vi "Insert an Empty Slot.vi"   [LabVIEW 2019]
doc: "Inserts an empty slot into an existing palette."
uses:
  <vilib>/Palette API/Palette Menu/Public Type Define/Palette type.ctl
  <vilib>/Palette API/Palette Menu/Public Type Define/Item.ctl
  <vilib>/Palette API/Palette Menu/Palette Menu.lvlib
panel:
  # "Overview: Demonstrates the use of the Palette Editing VIs to add an empty slot to an existing palette.\nInstructions:\n1. Make sure you have already run the Create New Palette.vi example.\n2. Run this VI. It will add an empty slot in the second position of the Functions > User Libraries > Palette API. See the block diagram for more information."
types:
  T1 = typedef "Palette Menu.lvlib/Palette type.ctl" = i32
  T2 = typedef "Palette Menu.lvlib/Palette Data.ctl" = cluster{"display name":string, "view format":T3, "palette width":i16, "items":T4, "256 color icon":picture, "B&W color icon":picture, "help information":T6, "palette description":string, "synchronize information":T7}
  T3 = typedef "Palette Menu.lvlib/View Format.ctl" = u16
  T4 = typedef "Palette Menu.lvlib/Items.ctl" = T5[]
  T5 = typedef "Palette Menu.lvlib/Item.ctl" = cluster{"item path":path, "library path":path, "use default lvlib palette":bool, "short name":string, "place VI contents":bool, "hide synchronized item":bool, "reserve spot for synch item":bool, "configure when placing VI contents":bool}
  T6 = typedef "Palette Menu.lvlib/Help Info.ctl" = cluster{"help tag":string, "help file path ":path}
  T7 = typedef "Palette Menu.lvlib/Synchronize Info.ctl" = cluster{"synchronize with directory":bool, "synchronize directory path":path}
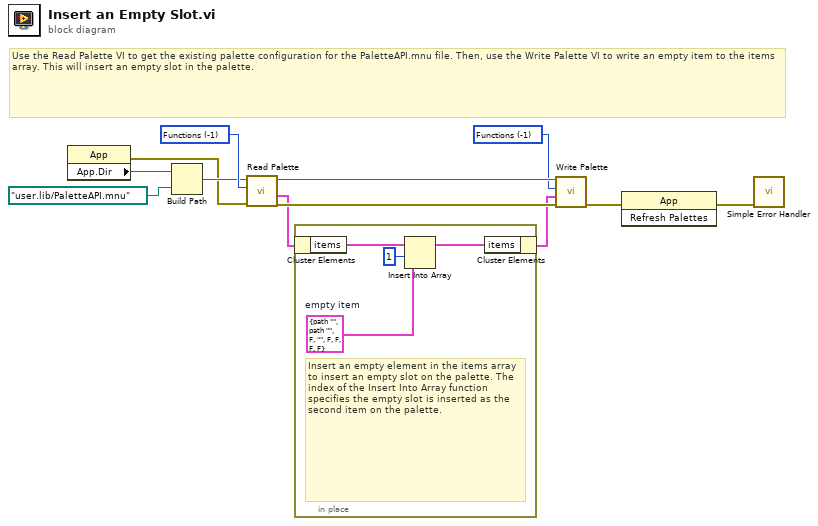
[diagram p0: block diagram]
diagram:
  w2 = T1 -1 items=["Functions"=-1, "Controls"=-2] ("palette type")
  w11 = T1 -1 items=["Functions"=-1, "Controls"=-2] ("palette type")
  # "Use the Read Palette VI to get the existing palette configuration for the PaletteAPI.mnu file. Then, use the Write Palette VI to write an empty item to the items array. This will insert an empty slot in the palette."
  n1 = property class="App"() -> (error out=w1:errorcluster, "App.Dir"=w5:path)  [unwired: 2 in, 1 out]
  n2 = Build Path(base path=w5, name or relative path=path "user.lib/PaletteAPI.mnu") -> (appended path=w8:path)
  n3 = call <vilib>:"Read Palette.vi"("error in (no error)"=w1, "palette type"=w11, "palette path"=w8) -> ("error out"=w10:errorcluster, "palette data"=w4:T2, "duplicate palette path"=w12:path)  [unwired: 1 in, 5 out]
  n4 = in-place {
    w13 = T5 {"item path"=path "", "library path"=path "", "use default lvlib palette"=FALSE, "short name"="", "place VI contents"=FALSE, "hide synchronized item"=FALSE, "reserve spot for synch item"=FALSE, "configure when placing VI contents"=FALSE}  # empty item
    # "Insert an empty element in the items array to insert an empty slot on the palette. The index of the Insert Into Array function specifies the empty slot is inserted as the second item on the palette."
    n5 = in-place-cluster #1(w4) -> ("items"=w15:T4)
    n6 = Insert Into Array(array=w15, index=1, new element=w13) -> (w14:T4)
    n7 = in-place-cluster #1("items"=w14) -> (w3:T2)
  }
  n8 = call <vilib>:"Write Palette.vi"("error in (no error)"=w10, "palette data"=w3, "palette type"=w2, "palette path"=w12) -> ("error out"=w7:errorcluster)  [unwired: 1 in, 6 out]
  n9 = invoke class="App" method="Refresh Palettes"(error in=w7) -> (error out=w6:errorcluster)  [unwired: 2 in, 2 out]
  n10 = call <vilib>:"Simple Error Handler.vi"("error in (no error)"=w6) -> ()  [unwired: 1 in, 8 out]
